vi "ADC_data_read.vi"(0 "Port Number":u16, 1 "Address":u32=49152 format="%x", 3 "Read_AVG ?":bool, 5 "Core Number":u16, 7 "Page":i32=1, 11 "error in (no error)":errorcluster, 13 "Lv_Samples":u32=16383) -> (4 "Read Data[]":u16[](array[numeric]), 6 "Read Data":dbl, 15 "error out":errorcluster)   [LabVIEW 2019]
uses:
  <userlib>/_TI-LA/Reusable/CCS/APIs/Data/Polymorphics/Read Data From Address - U16 Array.vi
  <userlib>/_TI-LA/Reusable/CCS/APIs/Data/Polymorphics/Read Data From Symbol - U32.vi
  <userlib>/_TI-LA/Reusable/CCS/APIs/CCS.lvlib
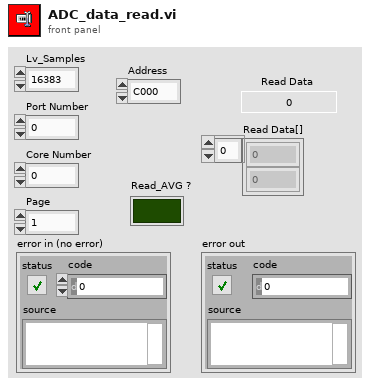
[diagram p1: front panel]
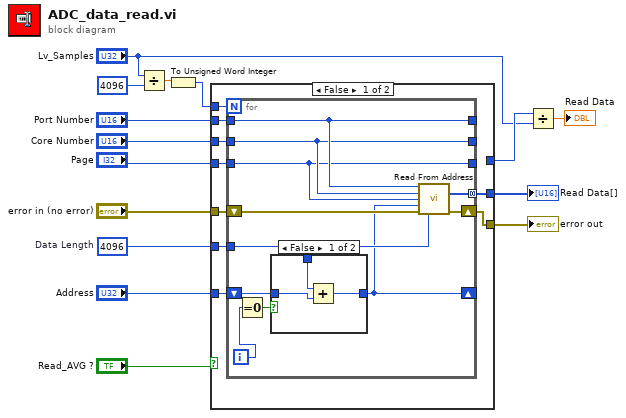
[diagram p0: block diagram]
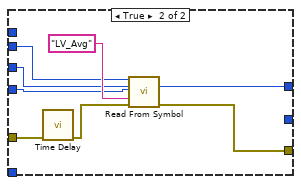
[diagram p3: hidden frame]
diagram:
  w10 = u32 4096  # Data Length
  n1 = Divide(x="Lv_Samples", y=u32 4096) -> (x/y=w2:dbl)
  n2 = To Unsigned Word Integer(number=w2) -> (unsigned 16bit integer=w1:u16)
  n3 = case shown="False" "Read_AVG ?" {
    tunnel: "Port Number" -> [w24 w44]
    tunnel: "Page" -> [w23 w42]
    tunnel: [w22 _] -> w13
    tunnel: "error in (no error)" -> [w21 w41]
    tunnel: "Core Number" -> [w20 w43]
    tunnel: w10 -> [w19 _]
    tunnel: "Address" -> [w18 _]
    tunnel: [_ w47] -> w6
    tunnel: [w17 w46] -> w5
    tunnel: w1 -> [w16 _]
    frame False {
      n4 = for {
        N: w16 -> [_]
        tunnel: w24 -> [w27]
        tunnel: w23 -> [w25]
        tunnel: [w34] -> w22 mode=concatenating
        tunnel: w20 -> [w26]
        tunnel: w19 -> [w29]
        shift-right: [w35] -> w17
        shift-left: w21 -> [w33]
        shift-right: [w28] -> _
        shift-left: w18 -> [w32]
        tunnel: [w27] -> _
        tunnel: [w26] -> _
        tunnel: [w25] -> _
        i -> [w30]
        n5 = Equal To 0?(x=w30) -> (x = 0?=w31:bool)
        n6 = case shown="False" w31 {
          tunnel: w32 -> [w36 w39]
          tunnel: [w38 w39] -> w28
          tunnel: w29 -> [w37 _]
          frame False {
            n7 = Add(x=w37, y=w36) -> (x+y=w38:u32)
          }
          frame True {
          }
        }
        n8 = call-poly <userlib>:"Read From Address.vi"("Port Number"=w27, "Core Number"=w26, "Page"=w25, "Address"=w28, "error in"=w33, "Data Length"=w29) -> ("Read Data[]"=w34:u16[], "error out"=w35:errorcluster)  [unwired: 6 in, 2 out]
      }
    }
    frame True {
      n9 = call "Time Delay"("error in (no error)"=w41) -> ("error out"=w40:errorcluster)  [unwired: 10 in]
      n10 = call-poly <userlib>:"Read From Symbol.vi"("Port Number"=w44, "Core Number"=w43, "Page"=w42, "Symbol Name"="LV_Avg", "error in"=w40) -> ("Read Data"=w47:u32, "error out"=w46:errorcluster)  [unwired: 7 in, 2 out]
    }
  }
  "error out" <- w5
  "Read Data[]" <- w13
  n11 = Divide(x=w6, y="Lv_Samples") -> (x/y=→"Read Data":dbl)
